vi "model.vi"() -> ()   [LabVIEW 2018]
uses:
  <vilib>/Analysis/3filter.llb/Filter Passband Type.ctl
  <vilib>/Analysis/3filter.llb/Butterworth Filter (DBL).vi
  <vilib>/Analysis/NI_AALBase.lvlib
panel:
  out "System Uptime":string
  out "Trend Chart":dbl(graph)
  out "lLOW alter led":bool
  out "Last Anomaly Time":string
  out "HIGH alter led":bool
  out "Variance":dbl
  out "Std dev":dbl
  out "RMS value":dbl
  out "Mean":dbl
  out "Filtered value indicator":dbl
  out "Current value indicator":dbl
  in  "STOP":bool
  # "ANALOG INSTRUMENT MONITORING SYSTEM"
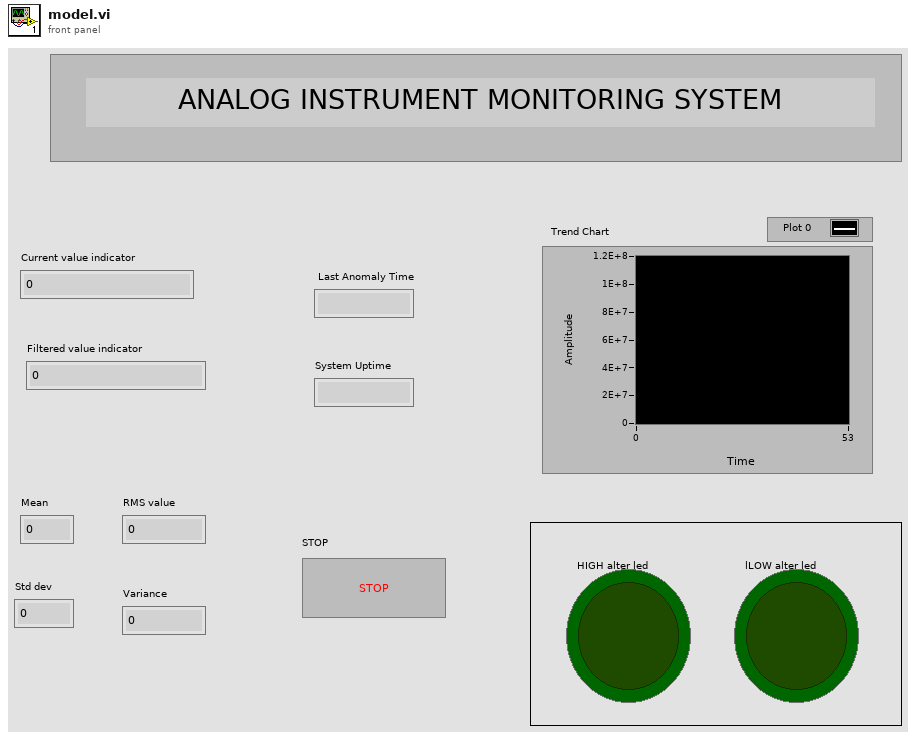
[diagram p1: front panel]
types:
  T1 = typedef "NI_AALBase.lvlib/Filter Passband Type.ctl" = enum32{"Lowpass", "Highpass", "Bandpass", "Bandstop"}
  T2 = enum16{"Standard", "Buffered", "CRLF", "Immediate"}
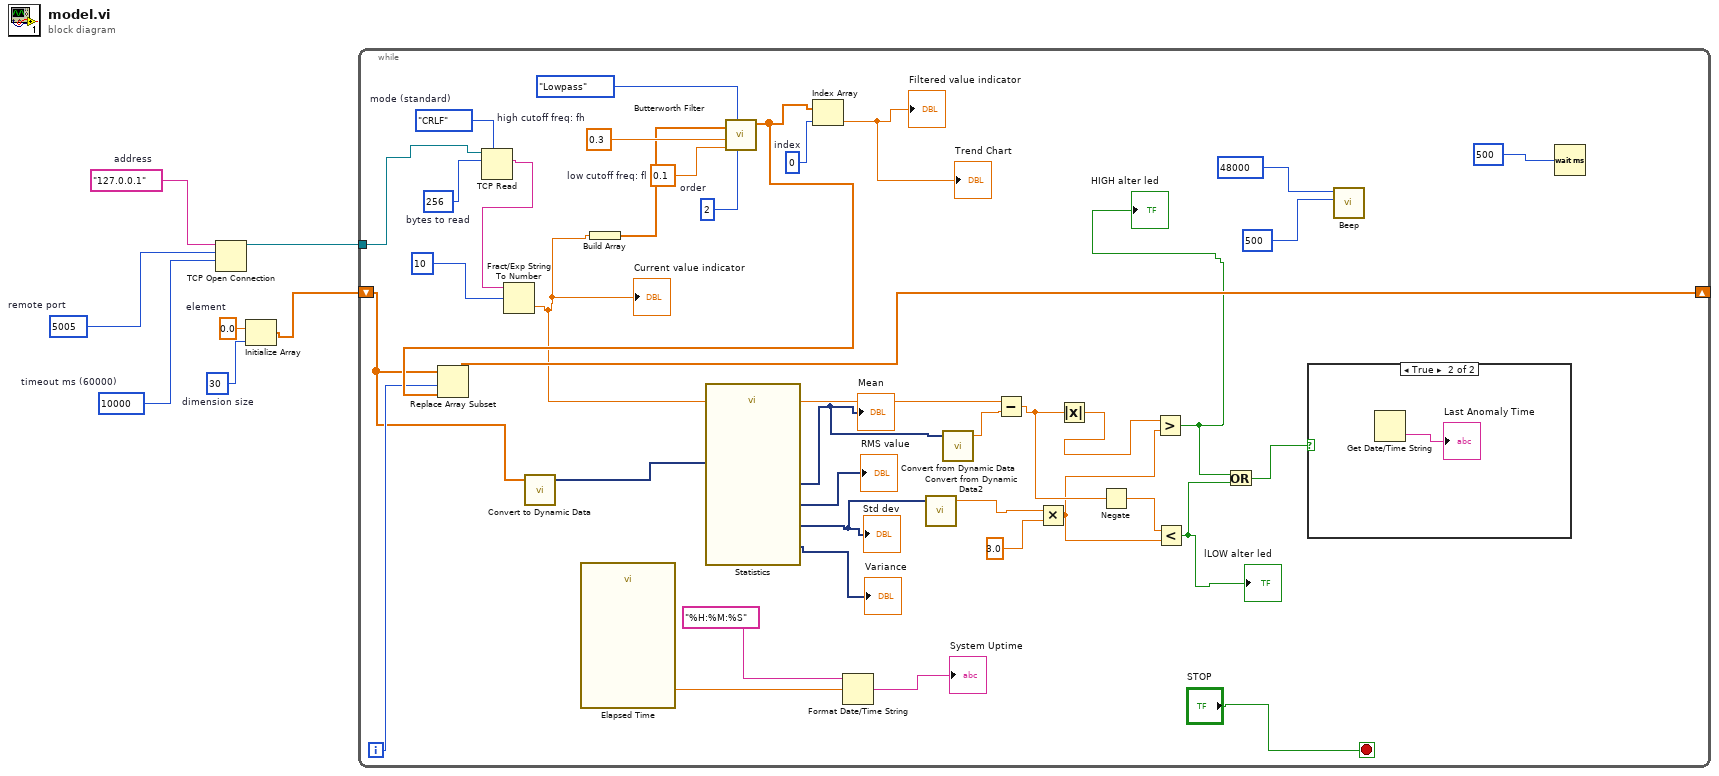
[diagram p0: block diagram]
diagram:
  w2 = 30  # dimension size
  w3 = 0.0  # element
  w4 = 10000  # timeout ms (60000)
  w6 = "127.0.0.1"  # address
  w7 = u16 5005  # remote port
  n1 = TCP Open Connection(address=w6, remote port or service name=w7, timeout ms (60000)=w4) -> (connection ID=w5:refnum<k5>)  [unwired: 2 in, 1 out]
  n2 = Initialize Array "Initialize Array"(w3, w2) -> (w1:dbl[])
  n3 = while {
    tunnel: w5 -> [w43]
    shift-right: [w35] -> _
    shift-left: w1 -> [w34]
    i -> [w36]
    stop <- "STOP" stop-if-true
    w38 = 0  # index
    w39 = 2  # order
    w40 = 0.1  # low cutoff freq: fl
    w41 = 0.3  # high cutoff freq: fh
    w45 = T2."CRLF"  # mode (standard)
    w46 = 256  # bytes to read
    n4 = TCP Read(connection ID=w43, bytes to read=w46, 7:w45) -> (data out=w11:string)  [unwired: 2 in, 2 out]
    n5 = Fract/Exp String To Number(string=w11, offset=10) -> (number=w8:dbl)  [unwired: 2 in, 1 out]
    "Current value indicator" <- w8
    n6 = call "Convert to Dynamic Data"("Array"=w34) -> ("Dynamic Data Type"=w33:dynamicdata)  [unwired: 3 in]
    n7 = call "Elapsed Time"() -> ("Elapsed Time (s)"=w18:dbl)  [unwired: 12 in, 7 out]
    n8 = Build Array "Build Array"(w8) -> (w10:dbl[])
    n9 = call "Statistics"("Signals"=w33) -> ("Variance"=→"Variance":dynamicdata, "Standard Dev"=w27:dynamicdata, "RMS"=→"RMS value":dynamicdata, "Arithmetic Mean"=w25:dynamicdata)  [unwired: 22 in, 1 out]
    "Mean" <- w25
    "Std dev" <- w27
    n10 = call-poly <vilib>:"Butterworth Filter.vi"("order"=w39, "filter type"=Filter_Passband_Type."Lowpass", "low cutoff freq: fl"=w40, "high cutoff freq: fh"=w41, "X"=w10) -> ("Filtered X"=w37:dbl[])  [unwired: 3 in, 1 out]
    n11 = Replace Array Subset "Replace Array Subset"(array=w34, new element=w37, index=w36) -> (w35:dbl[])
    n12 = Index Array "Index Array"(array=w37, index=w38) -> (element=→"Filtered value indicator" →"Trend Chart":dbl)
    n13 = Format Date/Time String(time format string (%c)="%H:%M:%S", seconds (now)=w18) -> (date/time string=→"System Uptime":string)  [unwired: 1 in]
    n14 = call "Convert from Dynamic Data2"("Dynamic Data Type"=w27) -> ("Scalar"=w28:dbl)  [unwired: 3 in]
    n15 = call "Convert from Dynamic Data"("Dynamic Data Type"=w25) -> ("Scalar"=w29:dbl)  [unwired: 3 in]
    n16 = Subtract(x=w8, y=w29) -> (x-y=w21:dbl)
    n17 = Multiply(x=w28, y=3.0) -> (x*y=w19:dbl)
    n18 = Absolute Value(x=w21) -> (abs(x)=w26:dbl)
    n19 = Negate(x=w21) -> (-x=w20:dbl)
    n20 = Greater?(x=w26, y=w19) -> (0:w14:bool)
    "HIGH alter led" <- w14
    n21 = Less?(x=w20, y=w19) -> (x < y?=w13:bool)
    "lLOW alter led" <- w13
    n22 = Or(x=w14, y=w13) -> (x .or. y?=w12:bool)
    n23 = case shown="True" w12 {
      frame False {
      }
      frame True {
        n24 = Get Date/Time String() -> (time string=→"Last Anomaly Time":string)  [unwired: 3 in, 1 out]
      }
    }
    n25 = call <vilib>:"Beep.vi"("duration (msec)"=u32 500, "frequency (Hz)"=u32 48000) -> ()  [unwired: 10 in]
    n26 = Wait (ms)(milliseconds to wait=u32 500) -> ()  [unwired: 1 out]
  }
